vi "setRampParameters.vi"(8 "error in (no error)":errorcluster, 10 "RampParameters":T1, 11 "RampToneAmplitudeDown in":refnum<class "RampToneAmplitudeDown.lvclass">) -> (0 "error out":errorcluster, 3 "RampToneAmplitudeDown out":refnum<class "RampToneAmplitudeDown.lvclass">)   [LabVIEW 2009, in "Tools.lvlib" / "Scripting.lvlib" / "RampToneAmplitudeDown.lvclass"]
uses:
  RampToneAmplitudeDown.lvclass
  SingleTone/SingleTone.lvclass
  RampTone/RampTone.lvclass
  ScriptEvent.lvclass
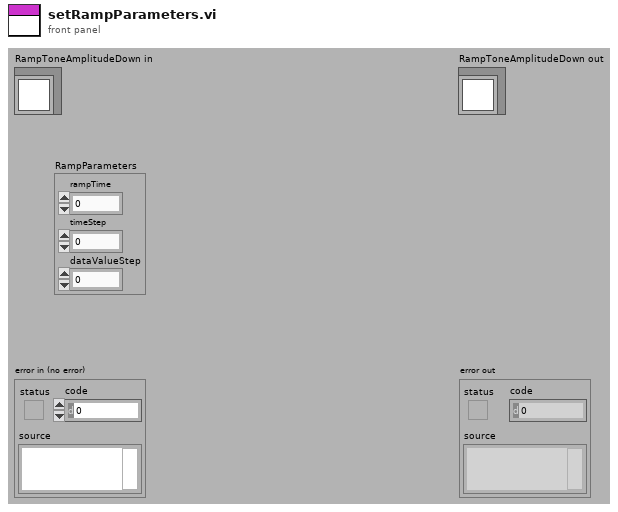
[diagram p1: front panel]
types:
  T1 = cluster{"rampTime":dbl, "timeStep":dbl, "dataValueStep":dbl}
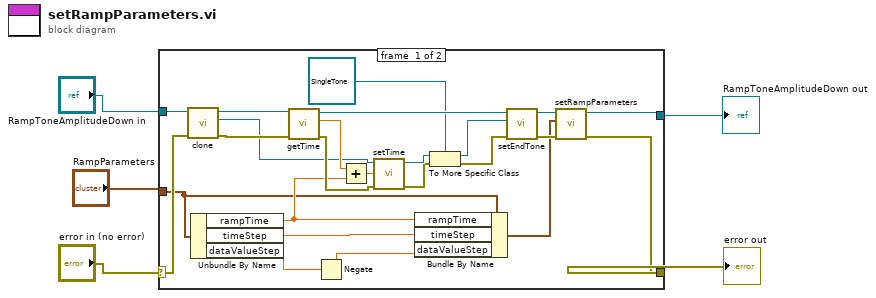
[diagram p0: block diagram]
diagram:
  n1 = case shown="No Error" "error in (no error)" {
    selector: "error in (no error)" -> [w23 w30]
    tunnel: "RampToneAmplitudeDown in" -> [w22 w31]
    tunnel: "RampParameters" -> [w14 _]
    tunnel: [w12 w30] -> w2
    tunnel: [w11 w31] -> w1
    frame #0 {
      n2 = call-dynamic "clone.vi"("error in (no error)"=w23, "SingleTone in"=w22) -> ("error out"=w24:errorcluster, "clone"=w21:refnum<class "ScriptEvent.lvclass">, "SingleTone out"=w25:refnum<class "RampToneAmplitudeDown.lvclass">)  [unwired: 7 in]
      n3 = Unbundle By Name(w14) -> ("rampTime"=w17:dbl, "timeStep"=w15:dbl, "dataValueStep"=w29:dbl)
      n4 = call "getTime.vi"("error in (no error)"=w24, "ScriptEvent.lvclass in"=w25) -> ("error out"=w26:errorcluster, "time"=w27:dbl, "ScriptEvent.lvclass out"=w20:refnum<class "RampToneAmplitudeDown.lvclass">)  [unwired: 7 in]
      n5 = Negate(x=w29) -> (-x=w16:dbl)
      n6 = Add(x=w27, y=w17) -> (x+y=w28:dbl)
      n7 = call "setTime.vi"("error in (no error)"=w26, "time"=w28, "ScriptEvent.lvclass in"=w21) -> ("error out"=w7:errorcluster, "ScriptEvent.lvclass out"=w9:refnum<class "ScriptEvent.lvclass">)  [unwired: 7 in]
      n8 = Bundle By Name(cluster=w14, "rampTime"=w17, "timeStep"=w15, "dataValueStep"=w16) -> (w13:T1)
      n9 = To More Specific Class(target class=refnum<class "SingleTone.lvclass"> refnum ("Tools.lvlib:Scripting.lvlib:SingleTone.lvclass"), reference=w9, error in=w7) -> (specific class reference=w8:refnum<class "SingleTone.lvclass">, error out=w6:errorcluster)
      n10 = call-dynamic "setEndTone.vi"("error in (no error)"=w6, "endTone"=w8, "RampTone.lvclass in"=w20) -> ("error out"=w19:errorcluster, "RampTone.lvclass out"=w18:refnum<class "RampToneAmplitudeDown.lvclass">)  [unwired: 7 in]
      n11 = call-parent "setRampParameters.vi"("error in (no error)"=w19, "RampParameters"=w13, "RampTone in"=w18) -> ("error out"=w12:errorcluster, "RampTone out"=w11:refnum<class "RampToneAmplitudeDown.lvclass">)  [unwired: 7 in]
    }
    frame #1 {
    }
  }
  "error out" <- w2
  "RampToneAmplitudeDown out" <- w1
